vi "Write UI Panel Launched Msg.vi"(10 "Chat Window UI Controller.lvlib:UI Panel Launched Msg.lvclass":refnum<class "UI Panel Launched Msg.lvclass">, 11 "Chat Window UI Controller in":refnum<class "Chat Window UI Controller.lvclass">) -> (3 "Chat Window UI Controller out":refnum<class "Chat Window UI Controller.lvclass">)   [LabVIEW 2014, in "Chat Window UI Controller.lvlib" / "Chat Window UI Controller.lvclass"]
uses:
  Chat Window UI Controller.lvclass
  Chat Window UI Controller Messages/UI Panel Launched Msg/UI Panel Launched Msg.lvclass
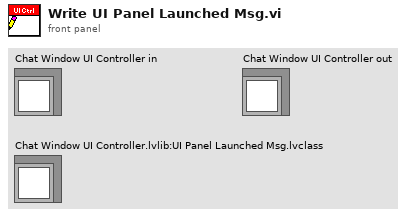
[diagram p1: front panel]
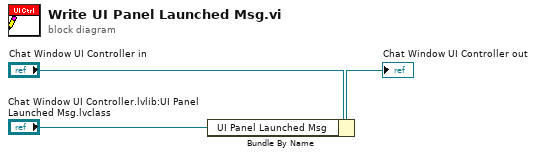
[diagram p0: block diagram]
diagram:
  n1 = Bundle By Name(cluster="Chat Window UI Controller in", "UI Panel Launched Msg"="Chat Window UI Controller.lvlib:UI Panel Launched Msg.lvclass") -> (→"Chat Window UI Controller out":refnum<class "Chat Window UI Controller.lvclass">)
